vi "_API_BINANCE_GET_AveragePriceFunction.vi"(0 "BinanceAPI in":refnum<class "BinanceAPI_.lvclass">, 5 "averagePriceFunction":cluster{"Symbol":string}, 11 "error in (no error)":errorcluster) -> (4 "BinanceAPI out":refnum<class "BinanceAPI_.lvclass">, 6 "Price (5 min average)":dbl format="%#.6g", 14 "Body":string, 15 "error out":errorcluster)   [LabVIEW 2022 SP3, in "BinanceAPI_.lvclass"]
doc: "https://binance-docs.github.io/apidocs/spot/en/#current-average-price"
uses:
  BinanceAPI_.lvclass
  BinanceAPI_.lvclass/BinanceAPI_.ctl
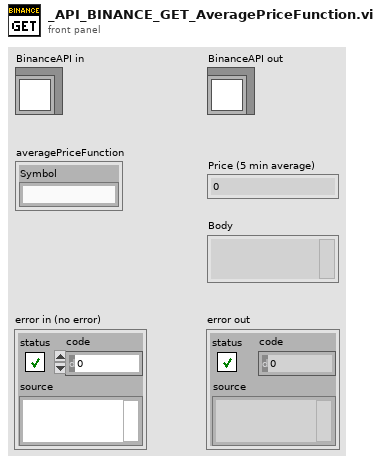
[diagram p1: front panel]
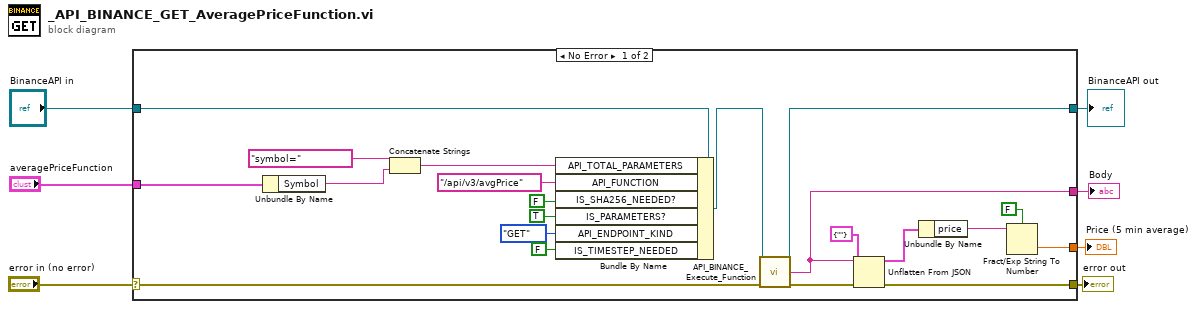
[diagram p0: block diagram]
diagram:
  n1 = case shown="No Error" "error in (no error)" {
    selector: "error in (no error)" -> [w16 w30]
    tunnel: [w14 w30] -> w6
    tunnel: [w17 w29] -> w2
    tunnel: "BinanceAPI in" -> [w26 w29]
    tunnel: "averagePriceFunction" -> [w24 _]
    tunnel: [w12 _] -> w4
    tunnel: [w8 _] -> w3
    frame No Error {
      n2 = Unbundle By Name(w24) -> ("Symbol"=w22:string)
      n3 = Concatenate Strings("symbol=" ("X-MBX-APIKEY: vmPUZE6mv9SD5VNHk4HlWFsOr6aKE2zvsw0MuIgwCIPy6utIco14y7Ju91duEh8A"), w22) -> (w21:string)
      n4 = Bundle By Name(cluster=w26, "API_TOTAL_PARAMETERS"=w21, "API_FUNCTION"="/api/v3/avgPrice" ("X-MBX-APIKEY: vmPUZE6mv9SD5VNHk4HlWFsOr6aKE2zvsw0MuIgwCIPy6utIco14y7Ju91duEh8A"), "IS_SHA256_NEEDED?"=FALSE, "IS_PARAMETERS?"=TRUE, "API_ENDPOINT_KIND"=enum16{"POST", "DELETE", "GET", "PUT"}."GET", "IS_TIMESTEP_NEEDED"=FALSE) -> (w18:refnum<class "BinanceAPI_.lvclass">)
      n5 = call "API_BINANCE_Execute_Function.vi"("BinanceAPI in"=w18, "error in (no error)"=w16) -> ("BinanceAPI out"=w17:refnum<class "BinanceAPI_.lvclass">, "Body"=w12:string, "error out"=w15:errorcluster)  [unwired: 9 in, 2 out]
      n6 = Unflatten From JSON(JSON string=w12, type and defaults=cluster{"price":string} {"price"=""}, error in (no error)=w15) -> (value=w11:cluster{"price":string}, error out=w14:errorcluster)  [unwired: 4 in]
      n7 = Unbundle By Name(w11) -> ("price"=w10:string)
      n8 = Fract/Exp String To Number(use system decimal point (T)=FALSE, string=w10) -> (number=w8:dbl)  [unwired: 2 in, 1 out]
    }
    frame Error {
    }
  }
  "error out" <- w6
  "Body" <- w4
  "Price (5 min average)" <- w3
  "BinanceAPI out" <- w2
